vi "Display Module - Detect IMAQ Ref Change.vi"(0 "Current Image Refs":T1[](array[typedef]), 11 "Previous Image Refs":T1[](array[typedef]), 13 "Previous Image Display Flags":bool[](array[boolean])) -> (4 "Current Image Refs (Dup)":T1[](array[typedef]), 8 "Change Detected":bool, 15 "Image Display Flags":bool[](array[boolean]))   [LabVIEW 2020]
uses:
  <vilib>/vision/Image Controls.llb/IMAQ Image.ctl
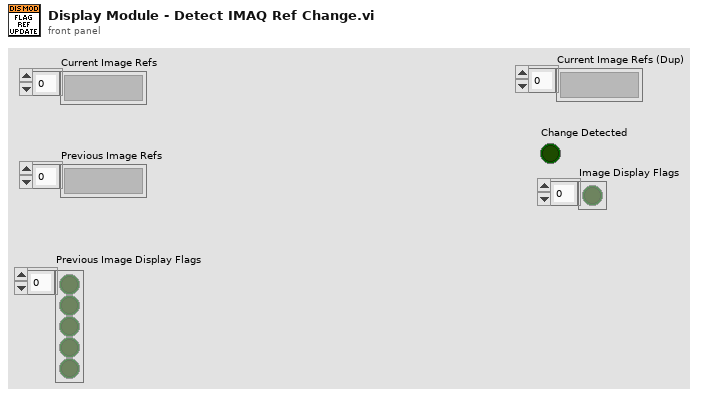
[diagram p1: front panel]
types:
  T1 = typedef "IMAQ Image.ctl" = refnum<image>
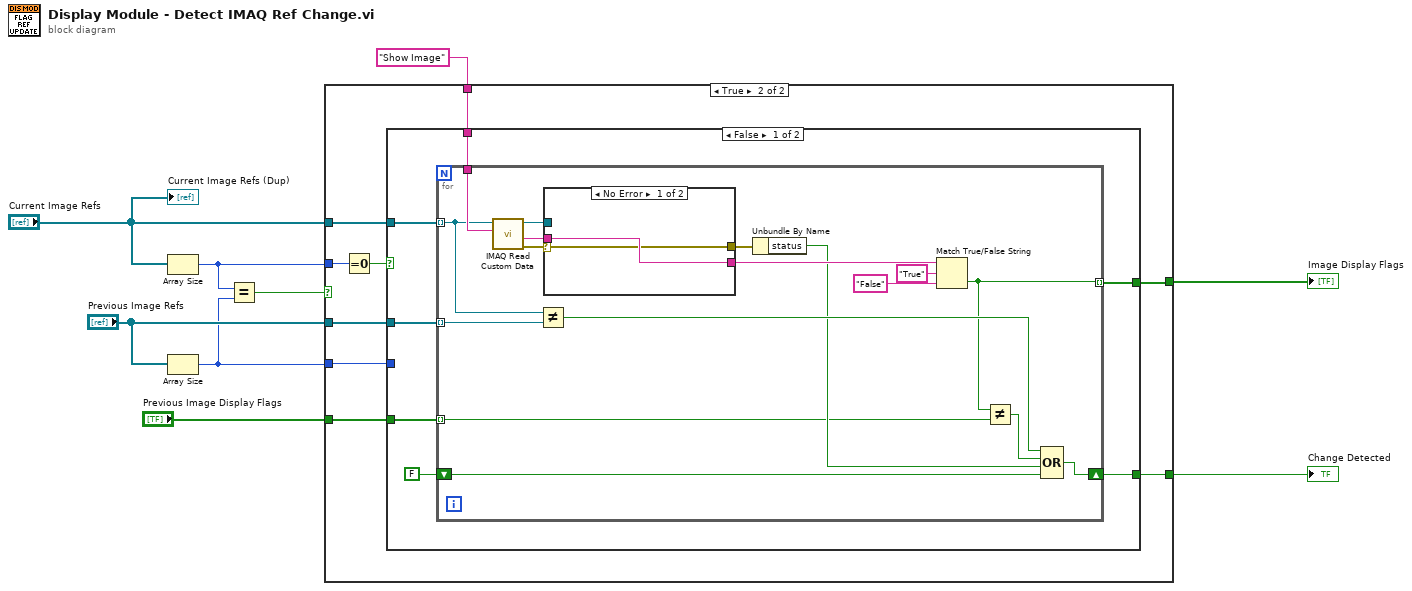
[diagram p0: block diagram]
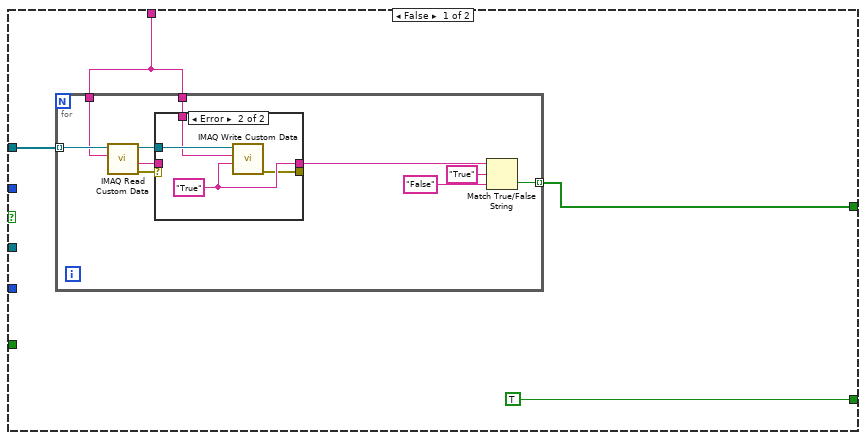
[diagram p2: hidden frame]
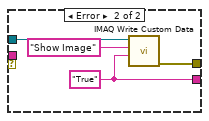
[diagram p4: hidden frame]
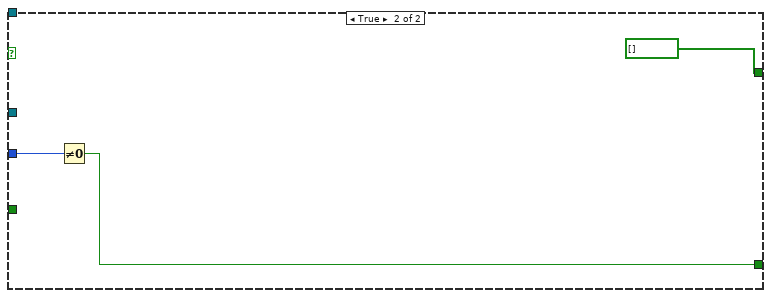
[diagram p5: hidden frame]
diagram:
  n1 = Array Size(array="Current Image Refs") -> (size(s)=w3:i32)
  n2 = Array Size(array="Previous Image Refs") -> (size(s)=w2:i32)
  n3 = Equal?(x=w3, y=w2) -> (x = y?=w9:bool)
  n4 = case shown="True" w9 {
    tunnel: "Current Image Refs" -> [w13 w38]
    tunnel: "Previous Image Refs" -> [_ w37]
    tunnel: [w12 w36] -> w7
    tunnel: [TRUE w34] -> w5
    tunnel: "Show Image" ("Key") -> [w10 w35]
    tunnel: w3 -> [_ w33]
    tunnel: w2 -> [_ w31]
    tunnel: "Previous Image Display Flags" -> [_ w30]
    frame False {
      n5 = for {
        tunnel: w13 -> [w21] mode=indexing
        tunnel: [w16] -> w12 mode=indexing
        tunnel: w10 -> [w15]
        tunnel: w10 -> [w14]
        n6 = call "IMAQ Read Custom Data"("Key"=w15, "Image"=w21) -> ("error out"=w23:errorcluster, "Custom Data Out"=w20:string, "Image (duplicate)"=w22:T1)  [unwired: 7 in]
        n7 = case shown="Error" w23 {
          selector: w23 -> [w24 _]
          tunnel: w22 -> [_ w29]
          tunnel: w20 -> [w25 _]
          tunnel: [w25 w28] -> w19
          tunnel: w14 -> [_ w27]
          tunnel: [w24 w26] -> _
          frame No Error {
          }
          frame Error {
            w28 = "True" ("Custom Data In")
            n8 = call "IMAQ Write Custom Data"("Custom Data In"=w28, "Key"=w27, "Image"=w29) -> ("error out"=w26:errorcluster)  [unwired: 7 in, 1 out]
          }
        }
        n9 = Match True/False String(2:"False" ("false string"), 3:"True" ("true string"), 4:w19) -> (0:w16:bool)  [unwired: 1 out]
      }
    }
    frame True {
      n10 = Equal To 0?(x=w33) -> (x = 0?=w32:bool)
      n11 = case shown="False" w32 {
        tunnel: w38 -> [w45 _]
        tunnel: w37 -> [w44 _]
        tunnel: [w43 bool[] []] -> w36
        tunnel: w35 -> [w42 _]
        tunnel: [w40 w70] -> w34
        tunnel: w31 -> [_ w71]
        tunnel: w30 -> [w39 _]
        frame False {
          n12 = for {
            tunnel: w45 -> [w54] mode=indexing
            tunnel: w44 -> [w55] mode=indexing
            tunnel: [w47] -> w43 mode=indexing
            tunnel: w42 -> [w56]
            shift-right: [w48] -> w40
            shift-left: FALSE -> [w52]
            tunnel: w39 -> [w46] mode=indexing
            n13 = call "IMAQ Read Custom Data"("Key"=w56, "Image"=w54) -> ("error out"=w62:errorcluster, "Custom Data Out"=w60:string, "Image (duplicate)"=w61:T1)  [unwired: 7 in]
            n14 = Not Equal?(x=w54, y=w55) -> (x != y?=w51:bool)
            n15 = case shown="No Error" w62 {
              selector: w62 -> [w63 _]
              tunnel: w61 -> [_ w68]
              tunnel: w60 -> [w64 _]
              tunnel: [w64 w66] -> w57
              tunnel: [w63 w65] -> w53
              frame No Error {
              }
              frame Error {
                w66 = "True" ("Custom Data In")
                n16 = call "IMAQ Write Custom Data"("Custom Data In"=w66, "Key"="Show Image", "Image"=w68) -> ("error out"=w65:errorcluster)  [unwired: 7 in, 1 out]
              }
            }
            n17 = Unbundle By Name(w53) -> ("status"=w49:bool)
            n18 = Match True/False String(2:"False" ("false string"), 3:"True" ("true string"), 4:w57) -> (0:w47:bool)  [unwired: 1 out]
            n19 = Not Equal?(x=w47, y=w46) -> (x != y?=w50:bool)
            n20 = Compound Arithmetic op=OR(w51, w50, w49, w52) -> (w48:bool)
          }
        }
        frame True {
          n21 = Not Equal To 0?(x=w71) -> (x != 0?=w70:bool)
        }
      }
    }
  }
  "Image Display Flags" <- w7
  "Change Detected" <- w5
  "Current Image Refs (Dup)" <- "Current Image Refs"
